vi "SaveOnFile2.vi"(1 "2D data":dbl[][](array[numeric]), 2 "1D data":dbl[](array[numeric]), 4 "file path (dialog if empty)":path) -> (7 "error file":errorcluster)   [LabVIEW 2019]
uses:
  <vilib>/Utility/file.llb/Write Delimited Spreadsheet (DBL).vi
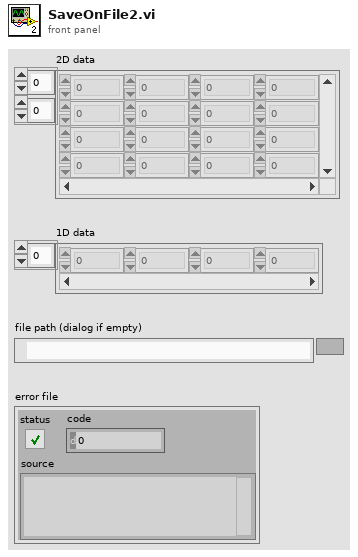
[diagram p1: front panel]
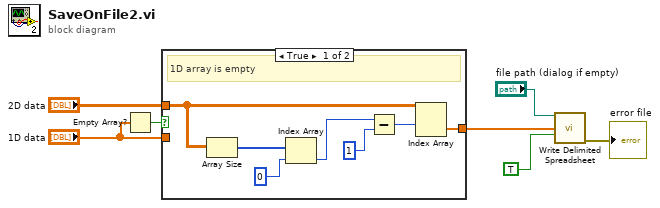
[diagram p0: block diagram]
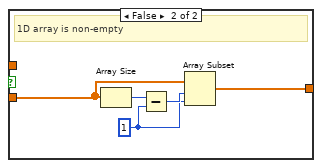
[diagram p2: hidden frame]
diagram:
  n1 = Empty Array?(array="1D data") -> (empty?=w4:bool)
  n2 = case shown="True" w4 {
    tunnel: "1D data" -> [_ w15]
    tunnel: "2D data" -> [w9 _]
    tunnel: [w8 w16] -> w1
    frame True {
      # "1D array is empty"
      n3 = Array Size(array=w9) -> (size(s)=w13:i32[])
      n4 = Index Array(array=w13, index=0) -> (element=w14:i32)
      n5 = Subtract(x=w14, y=1) -> (x-y=w12:i32)
      n6 = Index Array(array=w9, index (row)=w12) -> (element=w8:dbl[])  [unwired: 1 in]
    }
    frame False {
      w17 = 1 ("y")
      # "1D array is non-empty"
      n7 = Array Size(array=w15) -> (size(s)=w18:i32)
      n8 = Subtract(x=w18, y=w17) -> (x-y=w19:i32)
      n9 = Array Subset(array=w15, index=w19, length=w17) -> (w16:dbl[])
    }
  }
  n10 = call-poly <vilib>:"Write Delimited Spreadsheet.vi"("file path (dialog if empty)"="file path (dialog if empty)", "1D data"=w1, "append to file? (new file:F)"=TRUE) -> ("error out"=→"error file":errorcluster)  [unwired: 11 in, 1 out]
